vi "Read PARinitialised.vi"(8 "error in (no error)":errorcluster, 11 "PAR in":T1) -> (0 "error out":errorcluster, 2 "initialised":u8, 3 "PAR out":T1)   [LabVIEW 2019, in "Inputs.lvlib"]
uses:
  Inputs.lvlib
  Ctl/Param.ctl
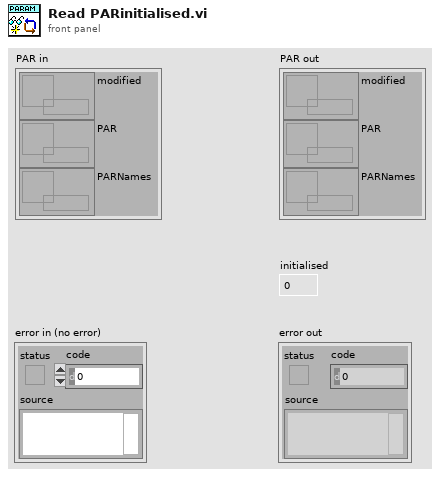
[diagram p1: front panel]
types:
  T1 = typedef "Inputs.lvlib/Param.ctl" = cluster{"modified":refnum<data-value>, "PAR":refnum<data-value>, "PARNames":refnum<data-value>}
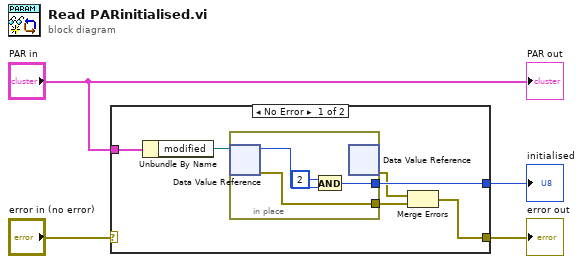
[diagram p0: block diagram]
diagram:
  n1 = case shown="No Error" "error in (no error)" {
    selector: "error in (no error)" -> [_ w15]
    tunnel: [w6 w15] -> w4
    tunnel: "PAR in" -> [w5 _]
    tunnel: [w9 _] -> w3
    frame No Error {
      n2 = Unbundle By Name(w5) -> ("modified"=w10:refnum<data-value>)
      n3 = in-place {
        in-place-border: [w14] -> w8
        in-place-border: [w12] -> w9
        n4 = in-place-dvr #1(w10) -> (w13:u8, w14:errorcluster)
        n5 = And(x=u8 2, y=w13) -> (x .and. y?=w12:u8)
        n6 = in-place-dvr #1() -> (w7:errorcluster)  [unwired: 1 in, 1 out]
      }
      n7 = Merge Errors(w7, w8) -> (w6:errorcluster)
    }
    frame Error {
    }
  }
  "error out" <- w4
  "initialised" <- w3
  "PAR out" <- "PAR in"
